vi "Transverse_Execute.vi"   [LabVIEW 2019]
uses:
  <vilib>/Rock Robotics/WPI/ThirdParty/Phoenix-LabVIEW/Motor Controller/Controls/CTRE_Phoenix_MotorControl_ControlMode.ctl
  Globals/Climb_Globals.vi
  Climb_Transverse_Control_States.ctl
  Climb_Transverse_Cluster.ctl
types:
  T1 = typedef "WPI_MotorControlDeviceRef.ctl" = cluster{"DeviceStatus":errorcluster, "Type":T2, "PWM":cluster{"PWM Channel":T3, "DeadBand":T4}, "CAN":cluster{"Device Number":u8, "SetOutput VI Ref":variant, "GetOutput VI Ref":variant, "Enable VI Ref":variant, "Disable VI Ref":variant, "Data":variant}, "Invert":bool, "DIO PWM":cluster{"PWM \"Enable\" Channel":T3, "DIOChannel":T5, "PWM Rate":dbl}}
  T2 = typedef "WPI_MotorControlType.ctl" = enum16{"PWM", "CAN", "DIO PWM"}
  T3 = typedef "FPGA_DIOPWMChannel.ctl" = enum8{"PWM 0", "PWM 1", "PWM 2", "PWM 3", "PWM 4", "PWM 5", "PWM 6", "PWM 7", "PWM 8", "PWM 9", "PWM MXP 0", "PWM MXP 1", "PWM MXP 2", "PWM MXP 3", "PWM MXP 4", "PWM MXP 5", "PWM MXP 6", "PWM MXP 7", "PWM MXP 8", "PWM MXP 9", "Invalid"}
  T4 = typedef "WPI_PWMDeadband.ctl" = cluster{"Name":string, "maxPositivePwm":i32, "minPositivePwm":i32, "centerPwm":i32, "maxNegativePwm":i32, "minNegativePwm":i32, "angularRange":u16}
  T5 = typedef "FPGA_DIOChannel.ctl" = enum8{"DIO 0", "DIO 1", "DIO 2", "DIO 3", "DIO 4", "DIO 5", "DIO 6", "DIO 7", "DIO 8", "DIO 9", "DIO MXP 0", "DIO MXP 1", "DIO MXP 2", "DIO MXP 3", "DIO MXP 4", "DIO MXP 5", "DIO MXP 6", "DIO MXP 7", "DIO MXP 8", "DIO MXP 9", "DIO MXP 10", "DIO MXP 11", "DIO MXP 12", "DIO MXP 13", "DIO MXP 14", "DIO MXP 15", "SPI Port CS1", "SPI Port CS2", "SPI Port CS3", "SPI Port MISO", "SPI Port MOSI", "Invalid"}
  T6 = typedef "Climb_Transverse_Cluster.ctl" = cluster{"Auto-Balance?":bool, "Transverse_Throttle":dbl, "Control_States":T7}
  T7 = typedef "Climb_Transverse_Control_States.ctl" = enum16{"No-Op", "Manual", "Auto-Balancing"}
  T8 = typedef "CTRE_Phoenix_MotorControl_ControlMode.ctl" = u16
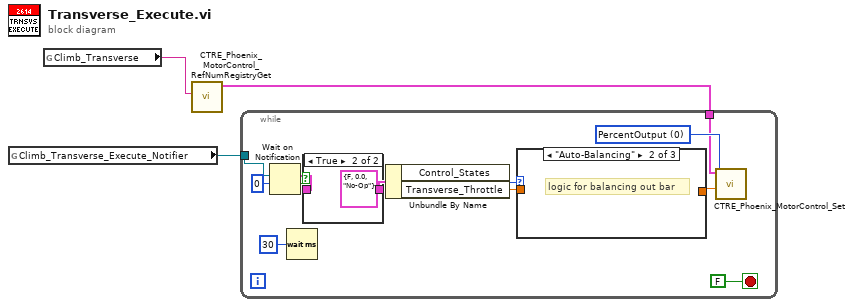
[diagram p0: block diagram]
diagram:
  n1 = global read "Climb_Globals.vi" "Climb_Transverse_Execute_Notifier"() -> (w3:refnum<notifier>)
  n2 = global read "Climb_Globals.vi" "Climb_Transverse"() -> (w2:string)
  n3 = call <vilib>:"CTRE_Phoenix_MotorControl_RefNumRegistryGet.vi"("refnum name"=w2) -> ("PhoenixMotorControlDevRef"=w1:T1)  [unwired: 9 in, 1 out]
  n4 = while {
    tunnel: w3 -> [w14]
    tunnel: w1 -> [w9]
    stop <- FALSE stop-if-true
    w10 = T8 0 items=["PercentOutput"=0, "Position"=1, "Velocity"=2, "Current"=3, "Follower"=5, "MotionProfile"=6, "MotionMagic"=7, "MotionProfileArc"=10, "Disabled"=15] ("Control Mode")
    n5 = Wait on Notification(notifier=w14, timeout in ms (-1)=0) -> (notification=w5:T6, timed out?=w6:bool)  [unwired: 2 in, 2 out]
    n6 = Wait (ms)(milliseconds to wait=u32 30) -> ()  [unwired: 1 out]
    n7 = case shown="True" w6 {
      tunnel: w5 -> [w16 _]
      tunnel: [w16 T6 {"Auto-Balance?"=FALSE, "Transverse_Throttle"=0.0, "Control_States"=enum."No-Op"} ("Climb_Transverse_Cluster")] -> w4
      frame False {
      }
      frame True {
      }
    }
    n8 = Unbundle By Name(w4) -> ("Control_States"=w13:T7, "Transverse_Throttle"=w12:dbl)
    n9 = case shown="\"Auto-Balancing\"" w13 {
      tunnel: w12 -> [_ _ w18]
      tunnel: [_ _ w18] -> w11
      frame "No-Op", Default {
      }
      frame "Auto-Balancing" {
        # "logic for balancing out bar"
      }
      frame "Manual" {
      }
    }
    n10 = call <vilib>:"CTRE_Phoenix_MotorControl_Set.vi"("Output"=w11, "Control Mode"=w10, "PhoenixMotorControlDevRef"=w9) -> ()  [unwired: 7 in, 2 out]
  }
